vi "dfd_FLP IIR I Transposed.vi"(7 "x":dbl format="%.2f", 8 "y states in":dbl[](array[numeric]) format="%.2f", 9 "x states in":dbl[](array[numeric]) format="%.2f", 10 "coefficients a":dbl[](array[numeric]) format="%.2f", 11 "coefficents b":dbl[](array[numeric]) format="%.2f") -> (0 "y states out":dbl[](array[numeric]) format="%.2f", 1 "x states out":dbl[](array[numeric]) format="%.2f", 2 "w":dbl, 3 "y":dbl format="%.2f")   [LabVIEW 2017, in "NI_DigFilter_FXP.lvlib"]
uses:
  <vilib>/addons/Digital Filter Design/NI_DigFilter_FXP.lvlib
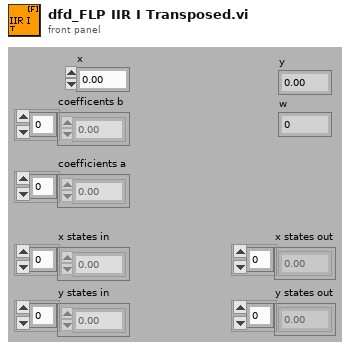
[diagram p1: front panel]
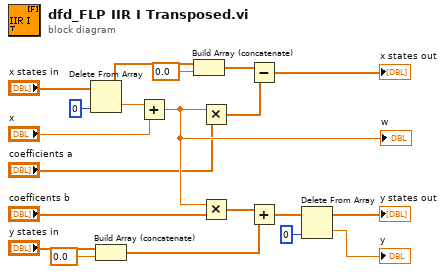
[diagram p0: block diagram]
diagram:
  n1 = Delete From Array(array="x states in", index=0) -> (deleted portion=w5:dbl, array with subset deleted=w14:dbl[])  [unwired: 1 in]
  n2 = Build Array (concatenate)("y states in", 0.0) -> (w8:dbl[])
  n3 = Add(x=w5, y="x") -> (x+y=w10:dbl)
  "w" <- w10
  n4 = Build Array (concatenate)(w14, 0.0) -> (w12:dbl[])
  n5 = Multiply(x=w10, y="coefficients a") -> (x*y=w11:dbl[])
  n6 = Multiply(x=w10, y="coefficents b") -> (x*y=w9:dbl[])
  n7 = Subtract(x=w12, y=w11) -> (x-y=→"x states out":dbl[])
  n8 = Add(x=w9, y=w8) -> (x+y=w7:dbl[])
  n9 = Delete From Array(array=w7, index=0) -> (deleted portion=→"y":dbl, array with subset deleted=→"y states out":dbl[])  [unwired: 1 in]
